vi "Robust Update.vi"(5 "condition":string, 7 "data":variant, 8 "error in (no error)":errorcluster, 9 "columns":string[](array[string])=["beh_stop_time"], 10 "table":string="behavior_traces ", 11 "AcquistionObject.lvclass":refnum<class "AcquistionObject.lvclass">) -> (0 "error out":errorcluster, 3 "AcquistionObject out":refnum<class "AcquistionObject.lvclass">)   [LabVIEW 2014, in "AcquisitionCoreObjects.lvlib" / "AcquistionObject.lvclass"]
uses:
  AcquistionObject.lvclass
  <vilib>/addons/database/NI_Database_API.lvlib
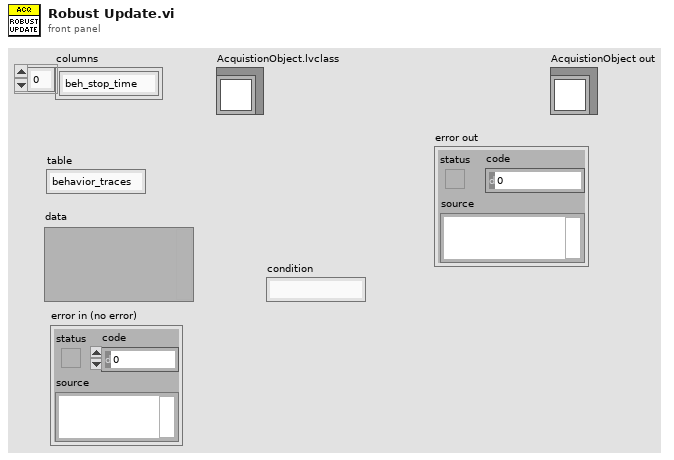
[diagram p1: front panel]
types:
  T1 = typedef "NI_Database_API.lvlib/Conn ObjectReference.ctl" = refnum<k1>
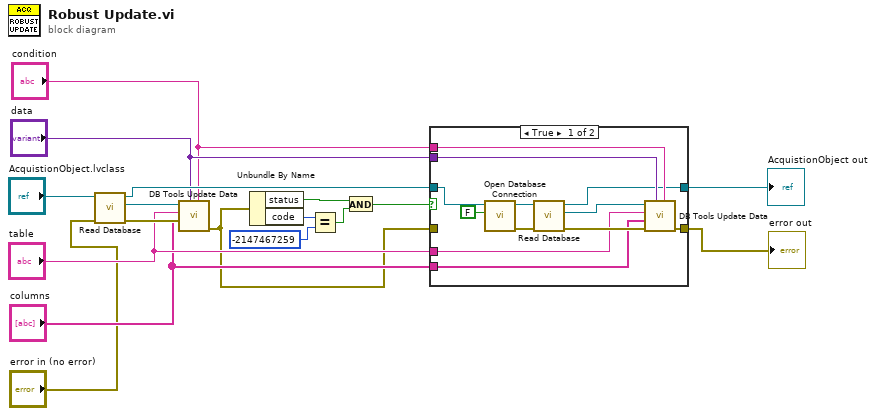
[diagram p0: block diagram]
diagram:
  n1 = call-dynamic "Read Database.vi"("error in (no error)"="error in (no error)", "AcquistionObject in"="AcquistionObject.lvclass") -> ("error out"=w16:errorcluster, "reference"=w12:T1, "AcquistionObject out"=w15:refnum<class "AcquistionObject.lvclass">)  [unwired: 7 in]
  n2 = call <vilib>:"DB Tools Update Data.vi"("condition"="condition", "data"="data", "error in (no error)"=w16, "columns"="columns", "table"="table", "connection reference"=w12) -> ("error out"=w1:errorcluster)  [unwired: 4 in, 1 out]
  n3 = Unbundle By Name(w1) -> ("status"=w3:bool, "code"=w6:i32)
  n4 = Equal?(x=w6, y=-2147467259) -> (x = y?=w4:bool)
  n5 = And(x=w3, y=w4) -> (x .and. y?=w2:bool)
  n6 = case shown="True" w2 {
    tunnel: w15 -> [w29 w31]
    tunnel: "table" -> [w25 _]
    tunnel: "columns" -> [w24 _]
    tunnel: "data" -> [w23 _]
    tunnel: "condition" -> [w22 _]
    tunnel: [w21 w30] -> w8
    tunnel: [w20 w31] -> w9
    tunnel: w1 -> [_ w30]
    frame True {
      n7 = call-dynamic "Open Database Connection.vi"("Initialize DatabaseQueue"=FALSE, "AcquistionObject in"=w29) -> ("error out"=w27:errorcluster, "AcquistionObject out"=w28:refnum<class "AcquistionObject.lvclass">)  [unwired: 8 in]
      n8 = call-dynamic "Read Database.vi"("error in (no error)"=w27, "AcquistionObject in"=w28) -> ("error out"=w26:errorcluster, "reference"=w19:T1, "AcquistionObject out"=w20:refnum<class "AcquistionObject.lvclass">)  [unwired: 7 in]
      n9 = call <vilib>:"DB Tools Update Data.vi"("condition"=w22, "data"=w23, "error in (no error)"=w26, "columns"=w24, "table"=w25, "connection reference"=w19) -> ("error out"=w21:errorcluster)  [unwired: 4 in, 1 out]
    }
    frame False {
    }
  }
  "AcquistionObject out" <- w9
  "error out" <- w8
